vi "roboRIO v1.0 Build MUX Configuration Encoder.vi"(11 "Channel":T4) -> (2 "Configuration Bitmask Array":bool[][](array[boolean]), 3 "Channel Reservation List":T1)   [LabVIEW 2021]
uses:
  <vilib>/myRIO/Common/Instrument Driver Framework/myRIO v1.0/Encoder/typedefs/Encoder Channels Enum.ctl
  <vilib>/myRIO/Common/Instrument Driver Framework/roboRIO v1.0/Resource Manager/typedefs/roboRIO v1.0 Channel Reservation List.ctl
  <vilib>/myRIO/Common/Instrument Driver Framework/roboRIO v1.0/Resource Manager/typedefs/roboRIO v1.0 Channel Reservation Info.ctl
  <vilib>/myRIO/Common/Instrument Driver Framework/roboRIO v1.0/Resource Manager/typedefs/roboRIO v1.0 Connector List.ctl
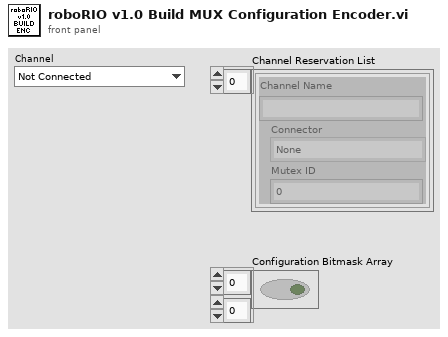
[diagram p1: front panel]
types:
  T1 = typedef "roboRIO v1.0 Channel Reservation List.ctl" = T2[]
  T2 = typedef "roboRIO v1.0 Channel Reservation Info.ctl" = cluster{"Channel Name":string, "Connector":T3, "Mutex ID":i32}
  T3 = typedef "roboRIO v1.0 Connector List.ctl" = enum32{"None", "ConnectorB", "ConnectorI2C", "ConnectorDIO", "ConnectorRSL", "ConnectorRELAY", "ConnectorAI", "ConnectorPWM", "ConnectorSPI"}
  T4 = typedef "Encoder Channels Enum.ctl" = enum16{"Not Connected", "C/ENC0", "C/ENC1", "A/ENC", "A/ENC0", "A/ENC1", "A/ENC2", "A/ENC3", "A/ENC4", "A/ENC5", "A/ENC6", "A/ENC7", "A/ENC8", "A/ENC9", "B/ENC", "B/ENC0", "B/ENC1", "B/ENC2", "B/ENC3", "B/ENC4", "B/ENC5", "B/ENC6", "B/ENC7", "B/ENC8", "B/ENC9", "DIO/ENC0", "DIO/ENC1", "DIO/ENC2", "DIO/ENC3", "DIO/ENC4"}
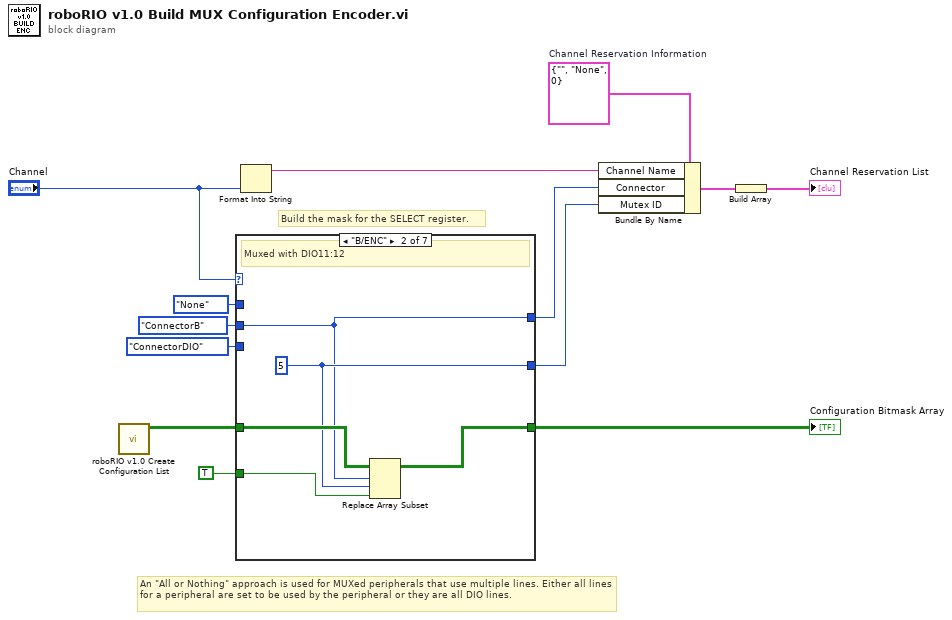
[diagram p0: block diagram]
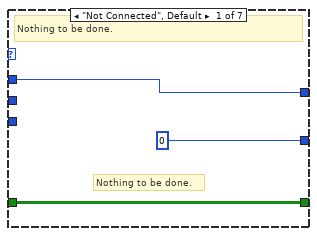
[diagram p2: hidden frame]
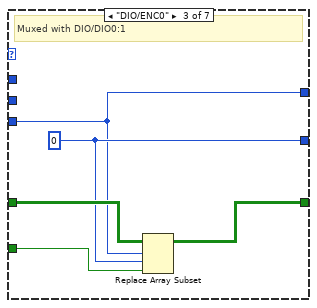
[diagram p3: hidden frame]
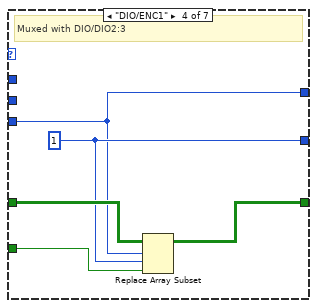
[diagram p4: hidden frame]
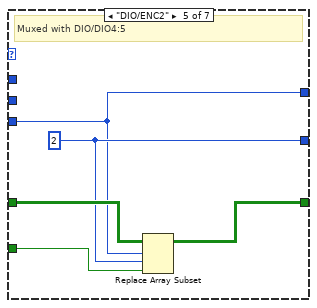
[diagram p5: hidden frame]
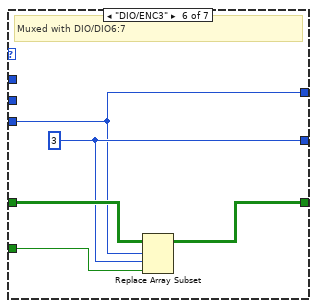
[diagram p6: hidden frame]
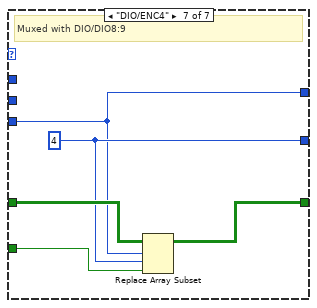
[diagram p7: hidden frame]
diagram:
  w6 = T2 {"Channel Name"="", "Connector"=enum."None", "Mutex ID"=0}  # Channel Reservation Information
  # "An \"All or Nothing\" approach is used for MUXed peripherals that use multiple lines. Either all lines for a peripheral are set to be used by the peripheral or they are all DIO lines."
  # "Build the mask for the SELECT register."
  n1 = call <vilib>:"roboRIO v1.0 Create Configuration List.vi"() -> ("Bitmask Array"=w3:bool[][])  [unwired: 11 in]
  n2 = case shown="\"B/ENC\"" "Channel" {
    tunnel: w3 -> [w16 w21 w26 w31 w36 w41 w46]
    tunnel: [w16 w20 w25 w30 w35 w40 w45] -> w10
    tunnel: roboRIO_v1.0_Connector_List."None" ("Connector List") -> [w15 _ _ _ _ _ _]
    tunnel: roboRIO_v1.0_Connector_List."ConnectorB" ("Connector List") -> [_ w17 _ _ _ _ _]
    tunnel: TRUE ("new element/subarray") -> [_ w19 w24 w29 w34 w39 w44]
    tunnel: roboRIO_v1.0_Connector_List."ConnectorDIO" ("Connector List") -> [_ _ w22 w27 w32 w37 w42]
    tunnel: [0 ("index") w18 w23 w28 w33 w38 w43] -> w1
    tunnel: [w15 w17 w22 w27 w32 w37 w42] -> w2
    frame "Not Connected", Default {
      # "Nothing to be done."
      # "Nothing to be done."
    }
    frame "B/ENC" {
      w18 = 5 ("index")
      # "Muxed with DIO11:12"
      n3 = Replace Array Subset(array=w21, new element=w19, index (row)=w17, index (col)=w18) -> (w20:bool[][])
    }
    frame "DIO/ENC0" {
      w23 = 0 ("index")
      # "Muxed with DIO/DIO0:1"
      n4 = Replace Array Subset(array=w26, new element=w24, index (row)=w22, index (col)=w23) -> (w25:bool[][])
    }
    frame "DIO/ENC1" {
      w28 = 1 ("index")
      # "Muxed with DIO/DIO2:3"
      n5 = Replace Array Subset(array=w31, new element=w29, index (row)=w27, index (col)=w28) -> (w30:bool[][])
    }
    frame "DIO/ENC2" {
      w33 = 2 ("index")
      # "Muxed with DIO/DIO4:5"
      n6 = Replace Array Subset(array=w36, new element=w34, index (row)=w32, index (col)=w33) -> (w35:bool[][])
    }
    frame "DIO/ENC3" {
      w38 = 3 ("index")
      # "Muxed with DIO/DIO6:7"
      n7 = Replace Array Subset(array=w41, new element=w39, index (row)=w37, index (col)=w38) -> (w40:bool[][])
    }
    frame "DIO/ENC4" {
      w43 = 4 ("index")
      # "Muxed with DIO/DIO8:9"
      n8 = Replace Array Subset(array=w46, new element=w44, index (row)=w42, index (col)=w43) -> (w45:bool[][])
    }
  }
  "Configuration Bitmask Array" <- w10
  n9 = Format Into String("Channel") -> (resulting string=w5:string)  [unwired: 3 in, 1 out]
  n10 = Bundle By Name(cluster=w6, "Channel Name"=w5, "Connector"=w2, "Mutex ID"=w1) -> (w7:T2)
  n11 = Build Array(w7) -> (→"Channel Reservation List":T2[])
